vi "TEMP-VI.vi"() -> ()   [LabVIEW 2026]
uses:
  <vilib>/MakerHub/LINX/Public/Peripherals/Analog/Analog Read 1 Chan.vi
  <vilib>/MakerHub/LINX/Public/Peripherals/Digital/Digital Read 1 Chan.vi
  <vilib>/MakerHub/LINX/Public/Peripherals/Analog/Analog Read N Chans.vi
  <vilib>/MakerHub/LINX/Public/Peripherals/Digital/Digital Read N Chans.vi
  <vilib>/MakerHub/LINX/Private/Local IO/LinxAnalogRead.vi
  <vilib>/MakerHub/LINX/Public/Utilities/Check Channel.vi
  <vilib>/MakerHub/LINX/Private/Local IO/LinxDigitalRead.vi
  <vilib>/MakerHub/LINX/Public/Utilities/Open Serial.vi
  <vilib>/MakerHub/LINX/Private/Utilties/Generate Error.vi
  <vilib>/MakerHub/LINX/LMH-LINX.lvlib
panel:
  out "23 Grados":bool
  out "40 Grados":bool
  out "INDICADOR":bool
  out "GRAFICA":i16(graph)
  out "Temperatura Indicador":dbl
  out "TEMPERATURA":dbl(slide) scale=0.0..100.0
  in  "Serial Port":refnum<visa-resource-name>="N/A"
  in  "STOP":bool
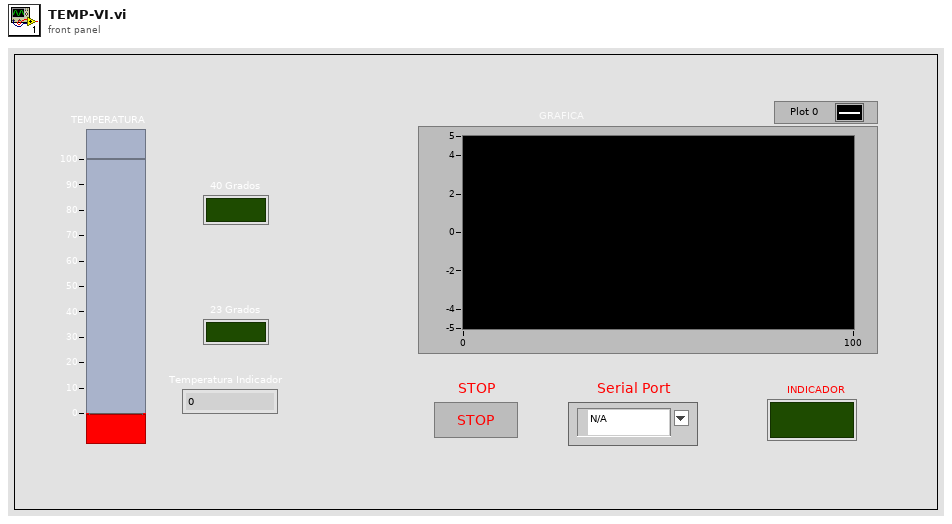
[diagram p1: front panel]
types:
  T1 = typedef "LMH-LINX.lvlib/LINX Ref.ctl" = cluster{"IO":T2, "Interface":T3, "LINX Device Config":T4}
  T2 = typedef "LMH-LINX.lvlib/Platform.ctl" = enum16{"Remote", "Local"}
  T3 = typedef "LMH-LINX.lvlib/Interface.ctl" = enum16{"Serial", "TCP"}
  T4 = typedef "LMH-LINX.lvlib/Device.lvlib/LINX Device Config.ctl" = cluster{"Interface":T3, "COM Port":refnum<visa-resource-name>, "TCP Configuration":T5, "Device Family":u8, "Device ID":u8, "Device Name":string, "TCP Ref":refnum<k5>, "Channels":T6}
  T5 = typedef "LMH-LINX.lvlib/Device.lvlib/TCP Config.ctl" = cluster{"IP Address":string, "Port":u16}
  T6 = typedef "LMH-LINX.lvlib/Channels.ctl" = cluster{"DI":u8[], "DO":u8[], "AI":u8[], "AO":u8[], "PWM":u8[], "QE":u8[], "UART":u8[], "I2C 2":u8[], "SPI":u8[], "CAN":u8[], "Servo":u8[], "AI Ref (V)":dbl, "AI Resolution (Bits)":u8, "AO Ref (V)":dbl, "AO Resolution (Bits)":u8}
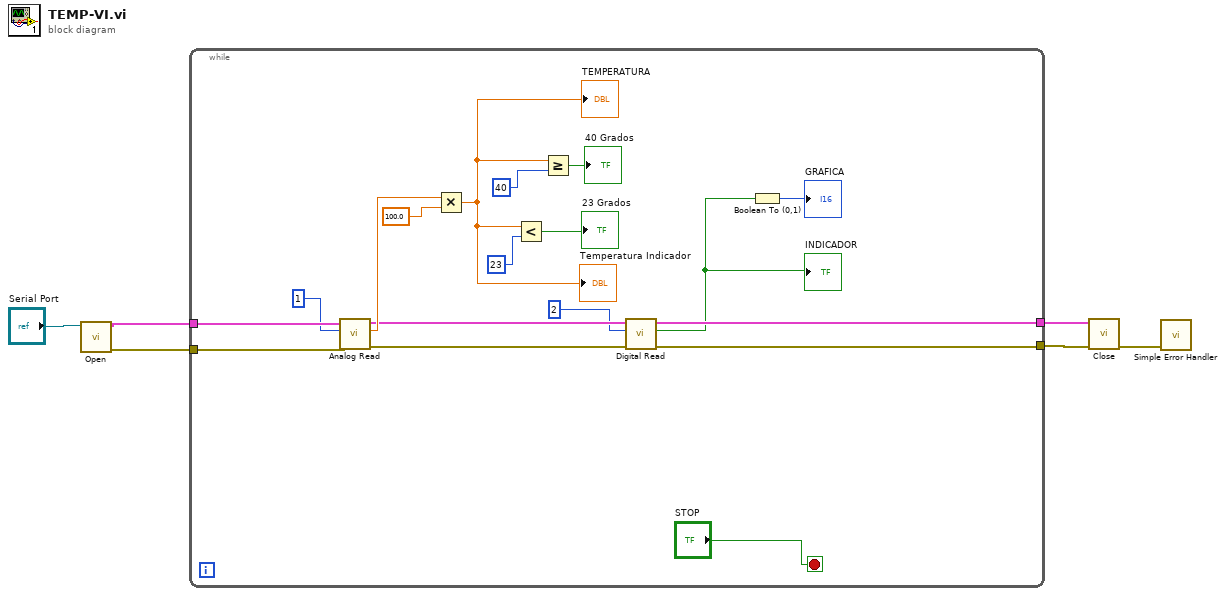
[diagram p0: block diagram]
diagram:
  n1 = call-poly <vilib>:"Open.vi"("Serial Port"="Serial Port") -> ("Error Out"=w4:errorcluster, "LINX Resource"=w5:T1)  [unwired: 8 in, 1 out]
  n2 = while {
    tunnel: w5 -> [w23]
    tunnel: w4 -> [w22]
    tunnel: [w16] -> w2
    tunnel: [w15] -> w1
    stop <- "STOP" stop-if-true
    n3 = call-poly <vilib>:"Analog Read.vi"("Error In"=w22, "Analog Channel"=u8 1, "LINX Resource"=w23) -> ("Error Out"=w17:errorcluster, "Voltage"=w20:dbl, "LINX Resource"=w18:T1)  [unwired: 5 in, 1 out]
    n4 = Multiply(x=w20, y=100.0) -> (x*y=w8:dbl)
    "TEMPERATURA" <- w8
    "Temperatura Indicador" <- w8
    n5 = Less?(x=w8, y=23) -> (x < y?=→"23 Grados":bool)
    n6 = Greater Or Equal?(x=w8, y=40) -> (x >= y?=→"40 Grados":bool)
    n7 = call-poly <vilib>:"Digital Read.vi"("Error In"=w17, "DI Channel"=u8 2, "LINX Resource"=w18) -> ("Error Out"=w15:errorcluster, "DI Value"=w12:bool, "LINX Resource"=w16:T1)  [unwired: 6 in]
    "INDICADOR" <- w12
    n8 = Boolean To (0,1)(Boolean=w12) -> (0, 1=→"GRAFICA":i16)
  }
  n9 = call <vilib>:"Close.vi"("Error In"=w1, "LINX Resource"=w2) -> ("Error Out"=w6:errorcluster)  [unwired: 9 in]
  n10 = call <vilib>:"Simple Error Handler.vi"("error in (no error)"=w6) -> ()  [unwired: 4 in, 5 out]
